vi "RT Loop - Acquire camera_test1.vi"(8 "rt fifo":refnum<k33>) -> (0 "error out":errorcluster)   [LabVIEW 2017]
uses:
  <vilib>/vision/Image Controls.llb/IMAQ Image.ctl
  <vilib>/userdefined/High Color/IMAQdx.ctl
  <vilib>/vision/driver/NI_Vision_Acquisition_Software.lvlib
panel:
  in  "error in (no error)":errorcluster
  out "error out 2":errorcluster
  in  "Stop Button":bool
  in  "Boolean":bool
  in  "y":bool
  out "Webcam":T1(plugin-control)
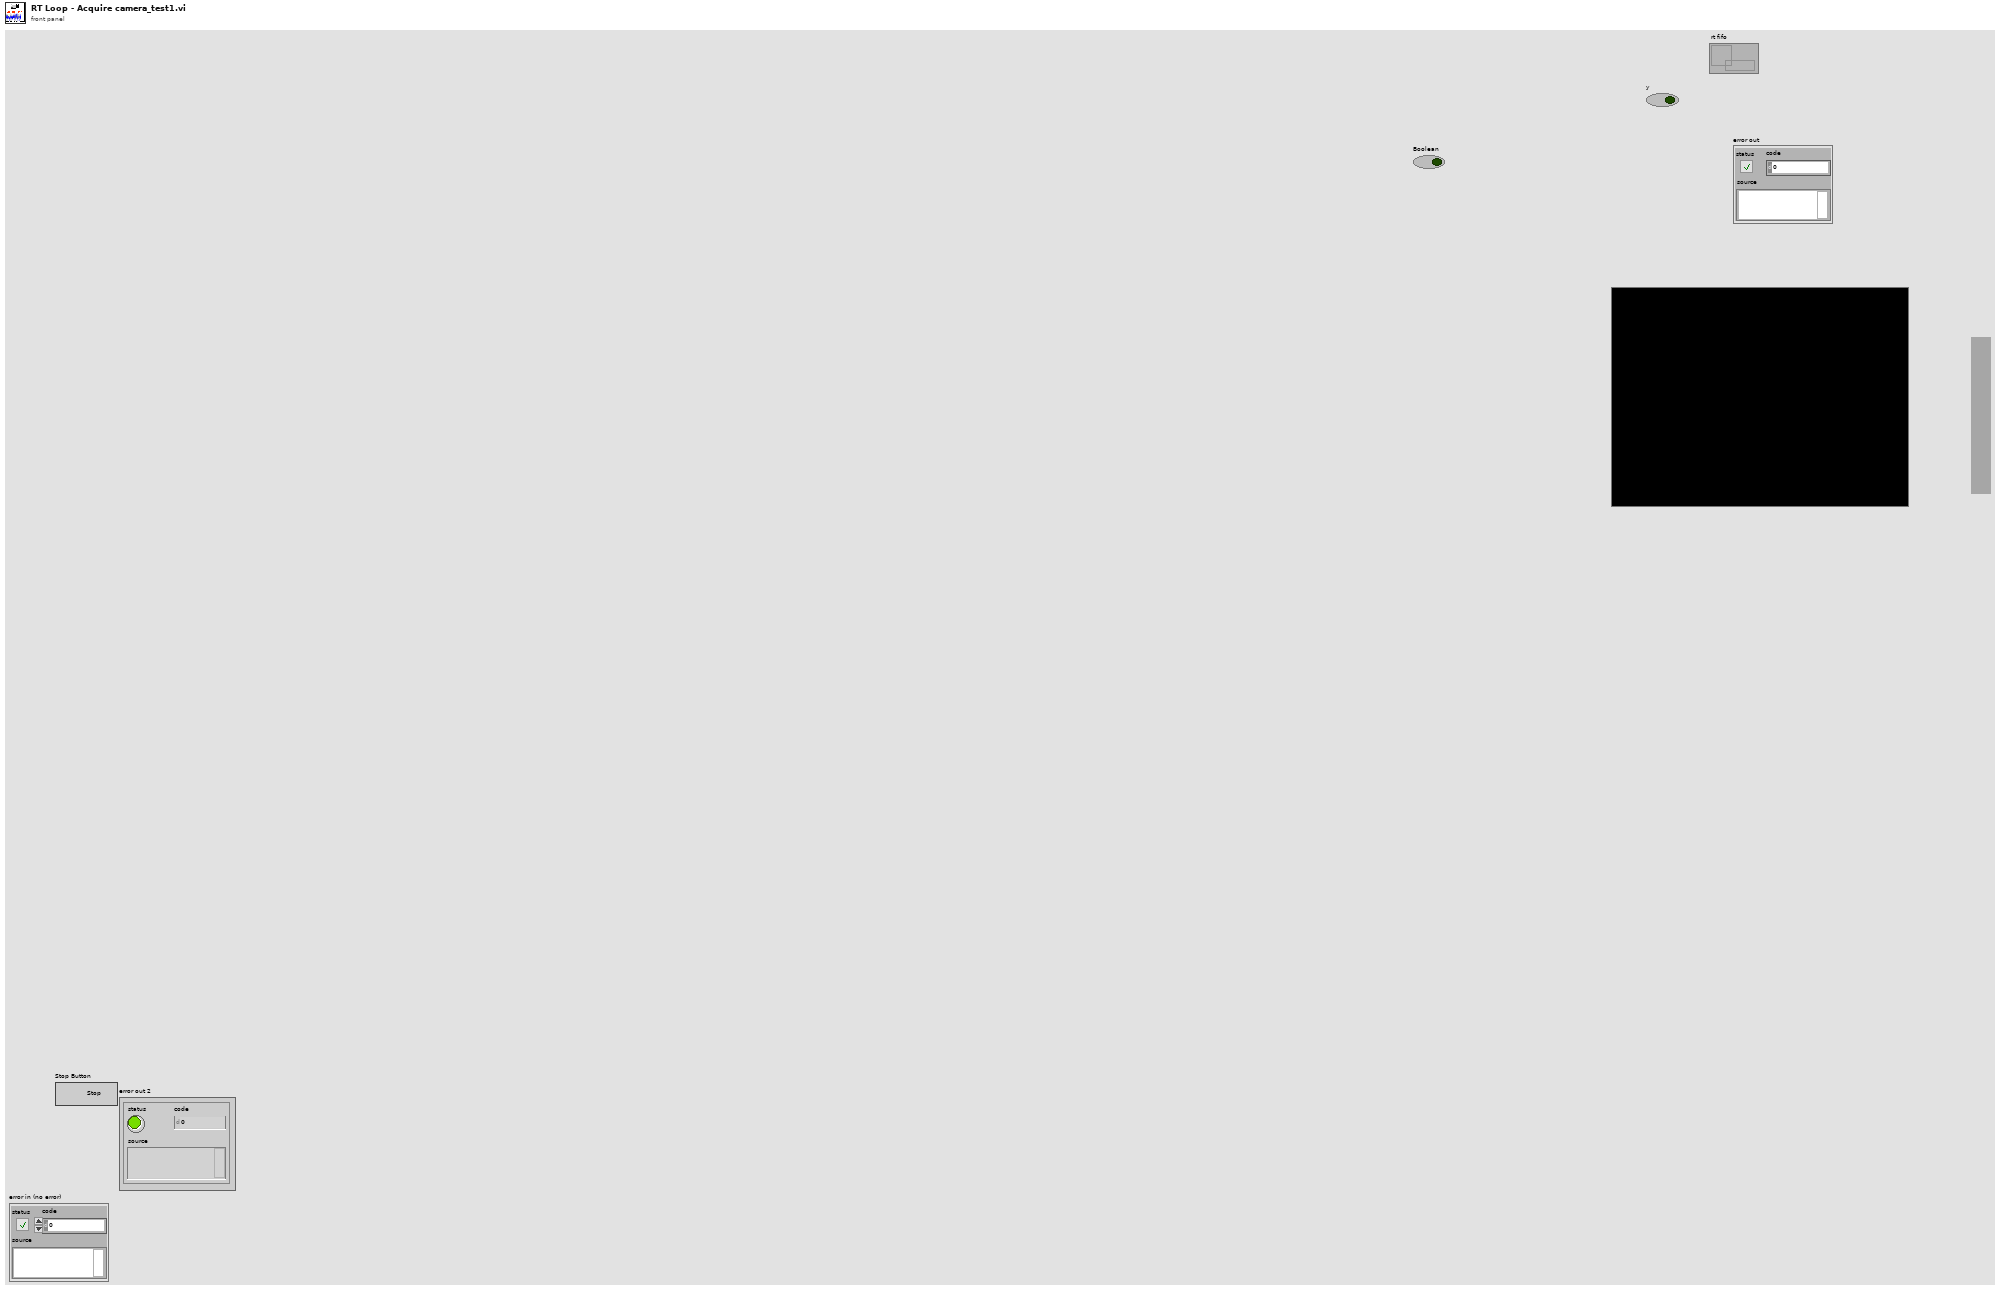
[diagram p1: front panel]
types:
  T1 = typedef "IMAQ Image.ctl" = refnum<image>
  T2 = typedef "IMAQdx.ctl" = refnum<k21>
  T3 = typedef "Image Type" = u32
  T4 = typedef "IMAQ AVI2 Refnum.ctl" = refnum<k20>
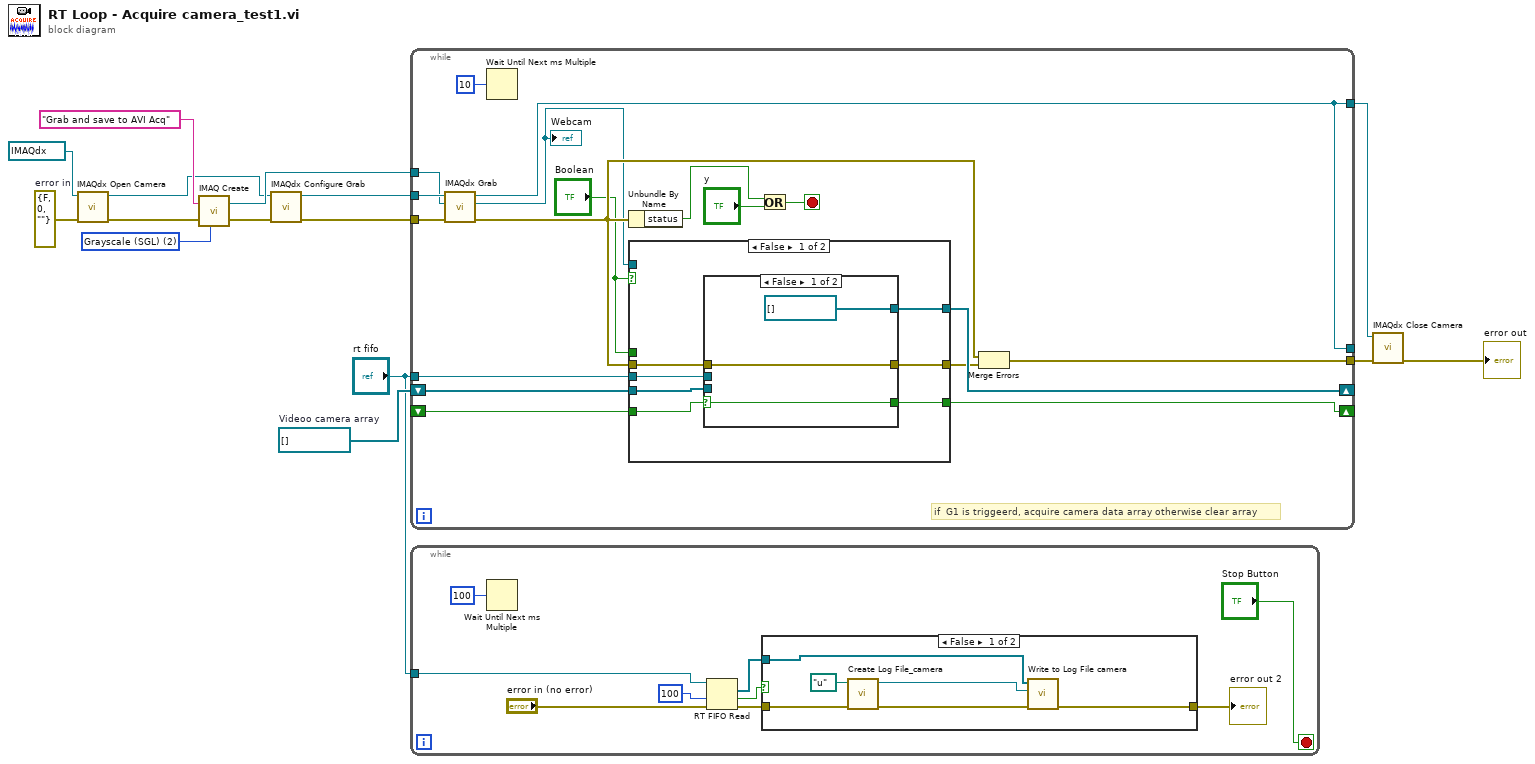
[diagram p0: block diagram]
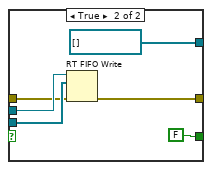
[diagram p3: hidden frame]
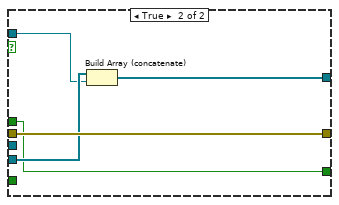
[diagram p4: hidden frame]
diagram:
  w2 = T1[] []  # Videoo camera array
  w8 = T3 2 items=["Grayscale (U8)", "Grayscale (I16)", "Grayscale (SGL)", "Complex (CSG)", "RGB (U32)", "HSL (U32)", "RGB (U64)", "Grayscale (U16)"] ("Image Type")
  w6 = errorcluster {"status"=FALSE, "code"=0, "source"=""}  # error in
  n1 = call <vilib>:"IMAQdx Open Camera.vi"("error in"=w6, "Session In"=T2 "cam0") -> ("error out"=w9:errorcluster, "Session Out"=w4:T2)  [unwired: 8 in]
  n2 = call "IMAQ Create"("Image Name"="Grab and save to AVI Acq", "Image Type"=w8, "error in (no error)"=w9) -> ("New Image"=w11:T1, "error out"=w12:errorcluster)  [unwired: 2 in]
  n3 = call <vilib>:"IMAQdx Configure Grab.vi"("error in"=w12, "Session In"=w4) -> ("error out"=w13:errorcluster, "Session Out"=w10:T2)  [unwired: 8 in]
  n4 = while {
    tunnel: [w27] -> _
    shift-right: [w26] -> _
    shift-left: w2 -> [w19]
    tunnel: "rt fifo" -> [w17]
    tunnel: w10 -> [w31]
    tunnel: w11 -> [w30]
    tunnel: w13 -> [w29]
    tunnel: [w27] -> w14
    tunnel: [w23] -> w3
    shift-right: [w21] -> _
    shift-left: _ -> [w20]
    stop <- w28 stop-if-true
    # "if  G1 is triggeerd, acquire camera data array otherwise clear array"
    n5 = call <vilib>:"IMAQdx Grab.vi"("error in"=w29, "Image In"=w30, "Session In"=w31) -> ("error out"=w24:errorcluster, "Image Out"=w22:T1, "Session Out"=w27:T2)  [unwired: 5 in, 1 out]
    "Webcam" <- w22
    n6 = Wait Until Next ms Multiple(millisecond multiple=u32 10 ("milliseconds to wait")) -> ()  [unwired: 1 out]
    n7 = Unbundle By Name(w24) -> ("status"=w32:bool)
    n8 = case shown="False" "Boolean" {
      tunnel: [w37 w51] -> w26
      tunnel: w17 -> [w38 _]
      tunnel: w24 -> [w35 w54]
      tunnel: [w34 w54] -> w25
      tunnel: w19 -> [w36 w53]
      tunnel: w22 -> [_ w52]
      tunnel: [w39 w50] -> w21
      tunnel: "Boolean" -> [_ w50]
      tunnel: w20 -> [w40 _]
      frame False {
        n9 = case shown="False" w40 {
          selector: w40 -> [w43 _]
          tunnel: [w43 FALSE] -> w39
          tunnel: w38 -> [_ w48]
          tunnel: w36 -> [_ w46]
          tunnel: [T1[] [] T1[] []] -> w37
          tunnel: w35 -> [w41 w45]
          tunnel: [w41 w44] -> w34
          frame False {
          }
          frame True {
            n10 = RT FIFO Write(0:w48, 1:w46, 3:w45) -> (11:w44:errorcluster)  [unwired: 2 in, 3 out]
          }
        }
      }
      frame True {
        n11 = Build Array (concatenate)(w53, w52) -> (w51:T1[])
      }
    }
    n12 = Or(x=w32, y="y") -> (x .or. y?=w28:bool)
    n13 = Merge Errors(w24, w25) -> (w23:errorcluster)
  }
  n14 = while {
    tunnel: "rt fifo" -> [w55]
    stop <- "Stop Button" stop-if-true
    n15 = Wait Until Next ms Multiple(millisecond multiple=u32 100 ("milliseconds to wait")) -> ()  [unwired: 1 out]
    n16 = RT FIFO Read(0:w55, 2:100 ("ms timeout (0)"), 3:"error in (no error)") -> (9:w58:T1[], 10:w62:bool, 11:w61:errorcluster)  [unwired: 1 in, 2 out]
    n17 = case shown="False" w62 {
      tunnel: w61 -> [w64 w70]
      tunnel: [w66 w70] -> w59
      tunnel: w58 -> [w67 _]
      frame False {
        n18 = call "Create Log File_camera.vi"("error in (no error)"=w64, "Acceleration Exceeded Log Folder"=path "u:/" ("file path (use dialog)")) -> ("error out"=w69:errorcluster, "AVI Refnum"=w68:T4)  [unwired: 8 in]
        n19 = call "Write to Log File camera.vi"("error in (no error)"=w69, "AVI Refnum in"=w68, "Array"=w67) -> ("error out"=w66:errorcluster)  [unwired: 7 in, 1 out]
      }
      frame True {
      }
    }
    "error out 2" <- w59
  }
  n20 = call <vilib>:"IMAQdx Close Camera.vi"("error in"=w3, "Session In"=w14) -> ("error out"=→"error out":errorcluster)  [unwired: 9 in]
